vi "Launch Tasks.vi"(8 "error in":errorcluster, 11 "Series Actor in":refnum<class "Series Actor.lvclass">) -> (0 "error out":errorcluster, 3 "Series Actor out":refnum<class "Series Actor.lvclass">)   [LabVIEW 2023, in "Series Actor.lvlib" / "Series Actor.lvclass"]
uses:
  Series Actor.lvclass
  Series Actor.lvclass/Series Actor.ctl
  Task/Task Actor/Task Actor/Task Actor.lvclass
  <vilib>/Utility/miscctls.llb/LVMapReplaceAction.ctl
  <vilib>/ActorFramework/Actor/Actor.lvclass
  a959e5df-b670-46ad-9029-43d23fac80d9.vi
  C:/Program Files/National Instruments/LabVIEW 2023/vi.lib/ActorFramework/Actor/Actor.lvclass
  D:/git/HAL/HAL GOOP4/Task/Task Actor/Task Actor/Task Actor.lvclass
  D:/git/HAL/HAL GOOP4/Task/ITask Actor/ITask Actor/ITask Actor.lvclass
  C:/Program Files/National Instruments/LabVIEW 2023/vi.lib/MGI/Panel Manager/Panel Actor/Panel Actor/Panel Actor.lvclass
  D:/git/HAL/HAL GOOP4/Series/Series Actor/Series Actor/Series Actor.lvclass
  D:/git/HAL/HAL GOOP4/Series/ISeries Actor/ISeries Actor/ISeries Actor.lvclass
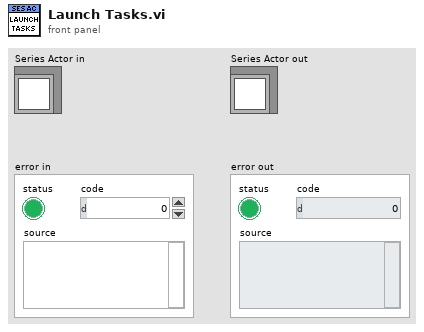
[diagram p1: front panel]
types:
  T1 = cluster{"Ident":string, "Class":string, "Point Idents":string[]}[]
  T2 = typedef "LVMapReplaceAction.ctl" = enum32{"Modify Entry only if found", "Add or Modify Entry", "Delete Entry"}
  T3 = map{string, refnum<class "Message Enqueuer.lvclass">}
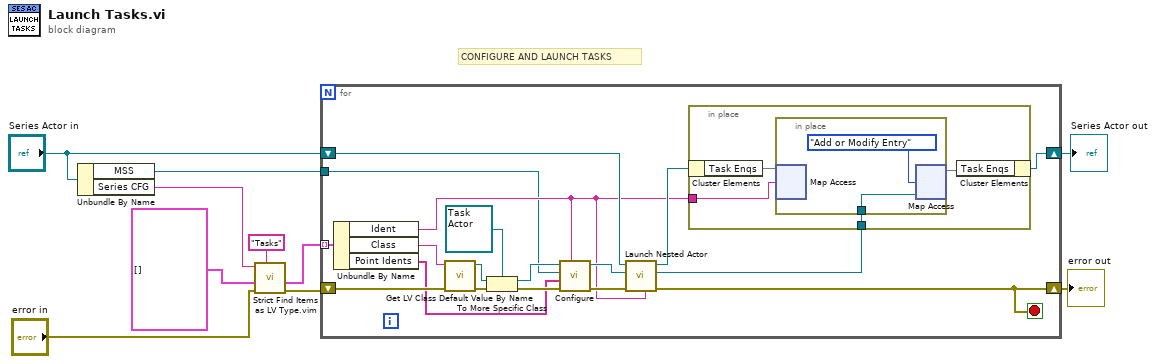
[diagram p0: block diagram]
diagram:
  # "CONFIGURE AND LAUNCH TASKS"
  n1 = Unbundle By Name("Series Actor in") -> ("MSS"=w5:refnum<class "Measure and Stimulus Subsystems.lvclass">, "Series CFG"=w6:string)
  n2 = call "Strict Find Items as LV Type.vim"("$Path or Item Name"="Tasks", "error in"="error in", "Data Type and Default Value"=T1 [] ("Tasks"), "JSON"=w6) -> ("error out"=w4:errorcluster, "Data out"=w3:T1)  [unwired: 6 in]
  n3 = for {
    tunnel: w3 -> [w25] mode=indexing
    shift-right: [w17] -> w9
    shift-left: w4 -> [w24]
    tunnel: w5 -> [w11]
    shift-right: [w20] -> w10
    shift-left: "Series Actor in" -> [w15]
    stop <- w17 stop-if-true
    n4 = Unbundle By Name(w25) -> ("Ident"=w12:string, "Class"=w23:string, "Point Idents"=w18:string[])
    n5 = call <vilib>:"Get LV Class Default Value By Name.vi"("error in (no error)"=w24, "class name"=w23) -> ("error out"=w28:errorcluster, "object"=w27:refnum<class>)  [unwired: 8 in]
    n6 = To More Specific Class(target class=refnum<class "Task Actor.lvclass"> refnum ("HAL GOOP4.lvlib:Task Base.lvclass"), reference=w27, error in=w28) -> (specific class reference=w22:refnum<class "Task Actor.lvclass">, error out=w21:errorcluster)
    n7 = call-dynamic "Configure.vi"("Task Ident"=w12, "error in"=w21, "Task-Point Idents"=w18, "MSS"=w11, "ITask Actor in"=w22) -> ("error out"=w19:errorcluster, "ITask Actor out"=w16:refnum<class "Task Actor.lvclass">)  [unwired: 5 in]
    n8 = call <vilib>:"Launch Nested Actor.vi"("Debug Alias"=w12, "error in (no error)"=w19, "Nested Actor"=w16, "Caller Actor in"=w15) -> ("error out"=w17:errorcluster, "Nested Actor's Enqueuer"=w13:refnum<class "Message Enqueuer.lvclass">, "Caller Actor out"=w14:refnum<class "Series Actor.lvclass">)  [unwired: 5 in]
    n9 = in-place {
      in-place-border: w13 -> [w31]
      in-place-border: w12 -> [w30]
      n10 = in-place-cluster #1(w14) -> ("Task Enqs"=w32:T3)
      n11 = in-place {
        in-place-border: w31 -> [w34]
        n12 = in-place-map #2(w32, w30) -> ()  [unwired: 1 in, 2 out]
        n13 = in-place-map #2(w34, LVMapReplaceAction."Add or Modify Entry" ("action")) -> (w29:T3)  [unwired: 2 out]
      }
      n14 = in-place-cluster #1("Task Enqs"=w29) -> (w20:refnum<class "Series Actor.lvclass">)
    }
  }
  "Series Actor out" <- w10
  "error out" <- w9
